vi "BRig_Host__Loop_Producer__tcp_System__Data_saveStateList.vi"(11 "input_filepath_storage":string) -> ()   [LabVIEW 2014]
uses:
  myRIO_BRig_RT__Case_Exp_stateList.ctl
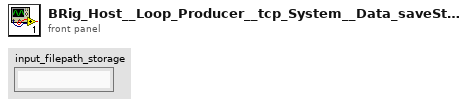
[diagram p1: front panel]
types:
  T1 = typedef "myRIO_BRig_RT__Case_Exp_stateList.ctl" = enum16{"Start1", "Start2", "Start3", "saveSettings1", "saveSettings2", "saveSettings3", "saveSettings4", "saveSettings_LC_ENL_l1", "saveSettings_LC_ENL_l2", "saveSettings_LC_Cue_l1", "saveSettings_LC_Cue_l2", "saveSettings6_LC_l1_Other", "SaveSettings6_LC_l2_Other", "setSettings_Audio", "setSettings_Laser", "initBlock_pre", "initBlock", "initBlock2", "initBlock_post", "initTrial_pre", "initTrial", "initTrial2", "initTrial3", "initTrial4", "initTrial_LC_ENL1", "initTrial_LC_Cue1", "initTrial_LC_Cue1_2", "initTrial_LC_Sel", "initTrial_post", "ENL1_pre", "ENL1", "ENL1_post", "ENL1Penalty_pre", "ENL1Penalty", "ENL2_pre", "ENL2", "ENL2Penalty_pre", "ENL2Penalty", "Cue1_pre", "Cue1", "Cue1_post", "Cue1Penalty_pre", "Cue1Penalty", "Cue2_pre", "Cue2", "Cue2Penalty_pre", "Cue2Penalty", "Selection_pre", "Selection", "Select_post", "SelectReward_pre", "SelectReward", "SelectRewardPost_pre", "SelectRewardPost", "SelectWrong_pre", "SelectWrong", "SelectWrong_post", "SelectTimeout_pre", "SelectTimeout", "SelectTimeout_post", "endTrial_pre", "endTrial1", "endTrial2", "endTrial3", "endTrial_post", "endBlock_pre", "endBlock", "endBlock_post", "endExp", "commConnect", "commUpload_pre", "commUpload_dataBlock", "commUpload_dataCurrent", "commUpload_dataExp", "commUpload_dataLC", "commUpload_dataTrial", "commUpload_post", "saveData_pre", "saveData_dataBlock", "saveData_dataCurrent", "saveData_dataExp", "saveData_dataLC", "saveData_dataTrial", "saveData_post", "empty_endBlock1", "empty_endBlock2", "empty_endTrial1", "empty_endTrial2", "empty_endTrial3", "empty_endTrial4", "empty_endTrial5", "dummyState", "dummyState_endBlock", "FreeReward_pre", "FreeReward", "FreeRewardPost_pre", "FreeRewardPost"}
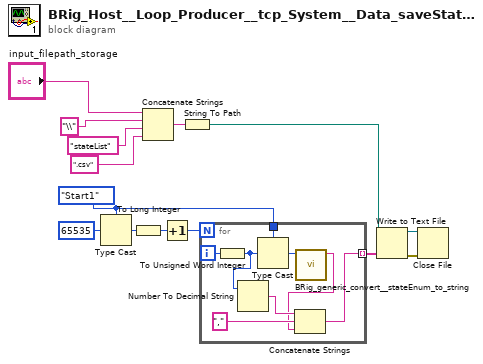
[diagram p0: block diagram]
diagram:
  w6 = myRIO_BRig_RT__Case_Exp_stateList."Start1" ("Enum")
  n1 = Type Cast(type=w6, x=u16 65535) -> (*(type *) &x=w9:T1)
  n2 = To Long Integer(number=w9) -> (32bit integer=w8:i32)
  n3 = Concatenate Strings("input_filepath_storage", "\\" ("string"), "stateList" ("input_fileName"), ".csv" ("string")) -> (w11:string)
  n4 = Increment(x=w8) -> (x+1=w7:i32)
  n5 = String To Path(string=w11) -> (path=w4:path)
  n6 = for {
    N: w7 -> [_]
    tunnel: w6 -> [w21]
    tunnel: [w15] -> w5 mode=indexing
    i -> [w20]
    n7 = To Unsigned Word Integer(number=w20) -> (unsigned 16bit integer=w17:u16)
    n8 = Number To Decimal String(number=w17) -> (decimal integer string=w18:string)  [unwired: 1 in]
    n9 = Type Cast(type=w21, x=w17) -> (*(type *) &x=w22:T1)
    n10 = call "BRig_generic_convert__stateEnum_to_string.vi"("input_stateEnum"=w22) -> ("output_str"=w16:string)  [unwired: 10 in]
    n11 = Concatenate Strings(w18, ",", w16) -> (w15:string)
  }
  n12 = Write to Text File(file (use dialog)=w4, text=w5) -> (refnum out=w3:refnum<file>, error out=w2:errorcluster)  [unwired: 2 in, 1 out]
  n13 = Close File(refnum=w3, error in=w2) -> ()  [unwired: 2 out]
